vi "Win32-Clear Always On Top.vi"(8 "error in (no error)":errorcluster, 11 "VI reference":refnum<vi>) -> (0 "error out":errorcluster)   [LabVIEW 2020]
uses:
  user32.dll
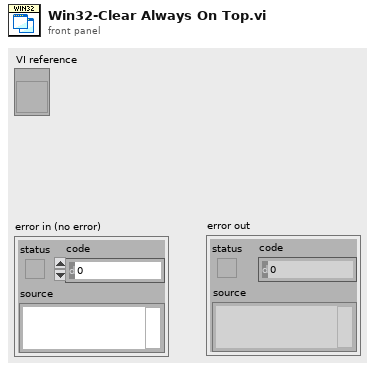
[diagram p1: front panel]
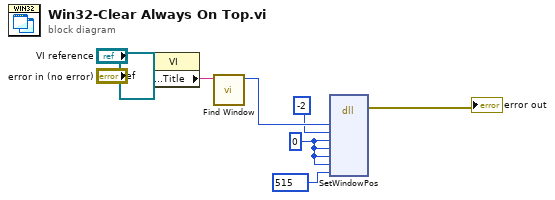
[diagram p0: block diagram]
diagram:
  (unwired) refnum<vi> refnum ("VI reference")
  w6 = 0 ("X")
  n1 = property class="VI"(reference="VI reference", error in="error in (no error)") -> ("Front Panel.Title"=w8:string)  [unwired: 2 out]
  n2 = call "Find Window.vi"("Window Name"=w8) -> ("Win32 Window Handle"=w7:i32)  [unwired: 9 in, 1 out]
  n3 = dll-call lib="user32.dll" fn="SetWindowPos"("hWnd"=w7, "hWndInsertAfter"=-2, "X"=w6, "Y"=w6, "cx"=w6, "cy"=w6, "uFlags"=u32 515) -> (error out=→"error out":errorcluster)  [unwired: 10 in, 2 out]
